vi "CRITERI RICERCA.vi"(6 "banco":i32=2, 8 "collaudi di confronto in":string[](array[string]), 9 "String 2":string="RICERCA COLLAUDI", 10 "Confronti?":bool) -> (0 "ANNULLA":bool=TRUE, 1 "collaudi di confronto":string[](array[string]), 2 "Collaudo selezionato":string, 3 "collaudi confronto descr":string[][](array[string]), 4 "Campi descrittivi confronto":string[](array[string]), 5 "Column Header Strings[]":string[](array[string])=["Banco", "Anno", "Numero", "CODICE", "Data_ora", "Anagrafica_cliente", "TIPO_PRODOTTO", "ARTICOLO", "GENERATORE_marca_generatore", "GENERATORE_marca_motore", "GENERATORE_marca_alternatore", "GENERATORE_matricola_alternatore", "GENERATORE_potenza_KVA", "GENERATORE_tensione_V", "GENERATORE_corrente", "GENERATORE_poli", "GENERATORE_giri", "GENERATORE_frequenza", "GENERATORE_tensione_eccitaz", "GENERATORE_corrente_eccitaz", "GENERICO_marca", "GENERICO_tipo", "GENERICO_matricola", "GENERICO_potenza_kW", "GENERICO_tensione_V", "GENERICO_corrente", "MOTOREac_marca", "MOTOREac_tipo", "MOTOREac_matricola", "MOTOREac_potenza_kW", "MOTOREac_poli", "MOTOREac_tensione_V", "MOTOREac_corrente", "MOTOREeex_marca", "MOTOREeex_tipo", "MOTOREeex_matricola", "MOTOREeex_poli", "MOTOREeex_potenza_kW", "MOTOREeex_tensione_V", "MOTOREeex_corrente", "MOTOREcc_marca", "MOTOREcc_tipo", "MOTOREcc_matricola", "MOTOREcc_potenza", "MOTOREcc_Tensione_Armatura", "MOTOREcc_Corrente_Armatura", "MOTOREcc_Tensione_campo", "MOTOREcc_Corrente_campo", "MOTOREcc_giri", "MOTOREcc_Tensione_dinamo", "POMPA_marca", "POMPA_tipo", "POMPA_matricola", "POMPA_poli", "POMPA_potenza_kw", "POMPA_tensione_V", "POMPA_corrente", "POMPAeex_marca", "POMPAeex_tipo", "POMPAeex_matricola", "POMPAeex_poli", "POMPAeex_potenza_kw", "POMPAeex_tensione_V", "POMPAeex_corrente", "TRASFORM_marca", "TRASFORM_tipo", "TRASFORM_matricola", "TRASFORM_potenza", "TRASFORM_tensione_primario", "TRASFORM_corrente_primario", "TRASFORM_tensione_secondario", "TRASFORM_corrente_secondario", "TRASFORM_gruppo_cei", "TRASFORM_VCC_percentuale", "collaudatore", "notes", "ESITO1", "ESITO2", "ESITO3", "ESITO4", "ESITO5", "ESITO6", "ESITO7", "ESITO8", "ESITO9", "ESITO10", "ESITO11", "ESITO12", "ESITO13", "ESITO14", "ESITO15", "NOTE_collaudo"], 7 "Campo descrittivo collaudo":string)   [LabVIEW 2019]
uses:
  <vilib>/Utility/miscctls.llb/LVRowAndColumnUnsignedTypeDef.ctl
  Global percorso impostazioni.vi
  <vilib>/Utility/file.llb/Read Delimited Spreadsheet (string).vi
  <vilib>/addons/database/Connection.llb/Conn Execute.vi
  <vilib>/addons/database/Recordset.llb/Rec Fetch Recordset Data (R).vi
  <vilib>/Utility/file.llb/Write Delimited Spreadsheet (string).vi
  <vilib>/addons/database/_DB Variant To Data/Database Variant To Data.xnode
  <vilib>/addons/database/NI_Database_API.lvlib
panel:
  in  "ARTICOLO":bool
  in  "TIPO":bool
  in  "CLIENTE":bool
  in  "ARTICOLO":string(combo)="MOTORE C.A."
  in  "TIPO PRODOTTO":string(combo)="3-MOTORE C.A."
  in  "ANAGRAFICA CLIENTE":string(combo)=" "
  out "Boolean":bool
  in  "ORDINA RISULTATI PER:":u16(ring)=5 items=["Banco", "Anno", "Numero", "CODICE", "Data_ora", "Anagrafica_cliente", "TIPO_PRODOTTO", "ARTICOLO", "GENERATORE_marca_generatore", "GENERATORE_marca_motore", "GENERATORE_marca_alternatore", "GENERATORE_matricola_alternatore", "GENERATORE_potenza_KVA", "GENERATORE_tensione_V", "GENERATORE_corrente", "GENERATORE_poli", "GENERATORE_giri", "GENERATORE_frequenza", "GENERATORE_tensione_eccitaz", "GENERATORE_corrente_eccitaz", "GENERICO_marca", "GENERICO_tipo", "GENERICO_matricola", "GENERICO_potenza_kW", "GENERICO_tensione_V", "GENERICO_corrente", "MOTOREac_marca", "MOTOREac_tipo", "MOTOREac_matricola", "MOTOREac_poli", "MOTOREac_potenza_kW", "MOTOREac_tensione_V", "MOTOREac_corrente", "MOTOREac_Frequenza", "MOTOREac_RPMnom", "MOTOREac_RPMmax", "MOTOREac_Costruttore", "MOTOREac_ModelloNr", "MOTOREac_TipoServizio", "MOTOREac_Design", "MOTOREac_ClasseIsol", "MOTOREac_Statore", "MOTOREac_Rotore", "MOTOREac_Note", "MOTOREeex_marca", "MOTOREeex_tipo", "MOTOREeex_matricola", "MOTOREeex_poli", "MOTOREeex_potenza_kW", "MOTOREeex_tensione_V", "MOTOREeex_corrente", "MOTOREcc_marca", "MOTOREcc_tipo", "MOTOREcc_matricola", "MOTOREcc_potenza", "MOTOREcc_Tensione_Armatura", "MOTOREcc_Corrente_Armatura", "MOTOREcc_Tensione_campo", "MOTOREcc_Corrente_campo", "MOTOREcc_giri", "MOTOREcc_Tensione_dinamo", "POMPA_marca", "POMPA_tipo", "POMPA_matricola", "POMPA_poli", "POMPA_potenza_kw", "POMPA_tensione_V", "POMPA_corrente", "POMPAeex_marca", "POMPAeex_tipo", "POMPAeex_matricola", "POMPAeex_poli", "POMPAeex_potenza_kw", "POMPAeex_tensione_V", "POMPAeex_corrente", "TRASFORM_marca", "TRASFORM_tipo", "TRASFORM_matricola", "TRASFORM_potenza", "TRASFORM_tensione_primario", "TRASFORM_corrente_primario", "TRASFORM_tensione_secondario", "TRASFORM_corrente_secondario", "TRASFORM_gruppo_cei", "TRASFORM_VCC_percentuale", "collaudatore", "notes", "ESITO1", "ESITO2", "ESITO3", "ESITO4", "ESITO5", "ESITO6", "ESITO7", "ESITO8", "ESITO9", "ESITO10", "ESITO11", "ESITO12", "ESITO13", "ESITO14", "ESITO15", "NOTE_collaudo"]
  out "transposed array":string[][](array[string])
  in  "Tab Control":T1(tab)=enum."OPZIONI"
  in  "COLLAUDI PER CARICAMENTO":i32(listbox)=-1
  in  "SELEZIONA COLLAUDO":bool
  in  "togli":bool
  in  "Lista collaudi":i32(listbox)=-1
  in  "COLLAUDI DI CONFRONTO":i32(listbox)=-1
  in  "AGGIUNGI CONFRONTO":bool
  in  "Fine":bool
  out "Campo descrittivo":string="Tipologia"
  in  "Scegli campo descrittivo":bool
  in  "Lista campi":i32(listbox)
  in  "salva Criteri":bool
  in  "gestione colonne":bool
  out "String":string
  out "filtri":bool[](array[boolean])=[TRUE, FALSE, FALSE, FALSE, FALSE, FALSE, FALSE]
  out "data":string[][](array[string])=[["1", "20", "1", "0", "", "3-MOTORE C.A.", "MOTORE C.A."], ["1", "20", "2", "0", "", "3-MOTORE C.A.", "MOTORE C.A."], ["1", "20", "3", "0", "", "3-MOTORE C.A.", "MOTORE C.A."], ["1", "20", "4", "0", "", "3-MOTORE C.A.", "MOTORE C.A."], ["1", "20", "5", "0", "", "3-MOTORE C.A.", "MOTORE C.A."], ["1", "20", "6", "0", "", "3-MOTORE C.A.", "MOTORE C.A."], ["1", "20", "7", "0", "", "3-MOTORE C.A.", "MOTORE C.A."], ["1", "20", "8", "0", "", "3-MOTORE C.A.", "MOTORE C.A."], ["1", "20", "9", "0", "", "3-MOTORE C.A.", "MOTORE C.A."], ["1", "20", "10", "0", "", "3-MOTORE C.A.", "MOTORE C.A."], ["1", "20", "11", "0", "", "3-MOTORE C.A.", "MOTORE C.A."], ["1", "20", "12", "0", "", "3-MOTORE C.A.", "MOTORE C.A."], ["1", "20", "13", "0", "", "3-MOTORE C.A.", "MOTORE C.A."], ["1", "20", "14", "0", "", "3-MOTORE C.A.", "MOTORE C.A."], ["1", "20", "15", "0", "", "3-MOTORE C.A.", "MOTORE C.A."], ["1", "20", "16", "0", "", "3-MOTORE C.A.", "MOTORE C.A."], ["1", "20", "17", "0", "", "3-MOTORE C.A.", "MOTORE C.A."], ["1", "20", "18", "0", "", "3-MOTORE C.A.", "MOTORE C.A."], ["1", "20", "19", "0", "", "3-MOTORE C.A.", "MOTORE C.A."], ["1", "20", "20", "0", "", "3-MOTORE C.A.", "MOTORE C.A."], ["1", "20", "21", "0", "", "3-MOTORE C.A.", ""], ["1", "20", "22", "0", "", "3-MOTORE C.A.", ""], ["1", "20", "23", "0", "", "3-MOTORE C.A.", ""], ["1", "20", "24", "0", "", "3-MOTORE C.A.", ""], ["1", "20", "25", "0", "", "3-MOTORE C.A.", ""], ["1", "20", "26", "0", "", "3-MOTORE C.A.", "MOTORE C.A."], ["1", "20", "27", "0", "", "3-MOTORE C.A.", "MOTORE C.A."], ["1", "20", "28", "0", "", "3-MOTORE C.A.", "MOTORE C.A."], ["1", "20", "29", "0", "", "3-MOTORE C.A.", "MOTORE C.A."], ["1", "20", "30", "0", "", "3-MOTORE C.A.", "MOTORE C.A."], ["1", "20", "31", "0", " ", "3-MOTORE C.A.", "MOTORE C.A."], ["1", "20", "32", "0", "", "3-MOTORE C.A.", "MOTORE C.A."], ["1", "20", "33", "0", " ", "3-MOTORE C.A.", "MOTORE C.A."], ["1", "20", "34", "0", " ", "3-MOTORE C.A.", "MOTORE C.A."], ["1", "20", "35", "0", " ", "3-MOTORE C.A.", "MOTORE C.A."], ["1", "20", "36", "0", " ", "3-MOTORE C.A.", "MOTORE C.A."], ["1", "20", "37", "0", " ", "3-MOTORE C.A.", "MOTORE C.A."], ["1", "20", "38", "0", " ", "3-MOTORE C.A.", "MOTORE C.A."], ["1", "20", "39", "0", " ", "3-MOTORE C.A.", "MOTORE C.A."], ["1", "20", "40", "0", " ", "3-MOTORE C.A.", "MOTORE C.A."], ["1", "20", "41", "0", " ", "3-MOTORE C.A.", "MOTORE C.A."], ["1", "20", "42", "0", " ", "3-MOTORE C.A.", "MOTORE C.A."], ["1", "20", "43", "0", " ", "3-MOTORE C.A.", " "], ["1", "20", "44", "0", " ", "3-MOTORE C.A.", " "], ["1", "20", "45", "0", " ", "3-MOTORE C.A.", " "], ["1", "20", "46", "0", " ", "3-MOTORE C.A.", " "], ["1", "20", "47", "0", " ", "3-MOTORE C.A.", " "], ["1", "20", "48", "0", " ", "3-MOTORE C.A.", " "], ["1", "20", "49", "0", " ", "3-MOTORE C.A.", " "], ["1", "20", "50", "0", " ", "3-MOTORE C.A.", " "], ["1", "20", "51", "0", " ", "3-MOTORE C.A.", " "], ["1", "20", "52", "0", "", "3-MOTORE C.A.", ""], ["1", "20", "53", "0", "", "3-MOTORE C.A.", ""], ["1", "20", "54", "0", "", "3-MOTORE C.A.", ""], ["1", "20", "55", "0", "", "3-MOTORE C.A.", ""], ["1", "20", "56", "0", "", "3-MOTORE C.A.", ""], ["1", "21", "1", "0", " ", "3-MOTORE C.A.", " "], ["2", "21", "1", "0", " ", "3-MOTORE C.A.", " "], ["1", "21", "2", "0", " ", "3-MOTORE C.A.", " "], ["1", "21", "3", "0", " ", "3-MOTORE C.A.", " "], ["1", "21", "4", "0", " ", "3-MOTORE C.A.", " "], ["1", "21", "5", "0", " ", "3-MOTORE C.A.", " "], ["2", "21", "2", "0", "", "3-MOTORE C.A.", ""], ["2", "21", "3", "0", "", "3-MOTORE C.A.", ""], ["2", "21", "4", "0", "", "3-MOTORE C.A.", ""], ["2", "21", "5", "0", "", "3-MOTORE C.A.", ""], ["2", "21", "6", "0", "", "3-MOTORE C.A.", ""], ["2", "21", "7", "0", "", "3-MOTORE C.A.", ""], ["2", "21", "8", "0", "", "3-MOTORE C.A.", ""], ["2", "21", "9", "0", "", "3-MOTORE C.A.", ""], ["1", "21", "6", "0", "", "3-MOTORE C.A.", ""], ["1", "21", "7", "0", "", "3-MOTORE C.A.", ""], ["1", "21", "8", "0", "", "3-MOTORE C.A.", ""], ["2", "21", "10", "0", "", "3-MOTORE C.A.", ""], ["2", "21", "12", "0", "", "3-MOTORE C.A.", ""], ["2", "21", "13", "0", "", "3-MOTORE C.A.", ""], ["2", "21", "15", "0", "", "3-MOTORE C.A.", ""], ["2", "21", "14", "0", "", "3-MOTORE C.A.", ""], ["1", "21", "9", "0", "", "3-MOTORE C.A.", "MOTORE C.A."], ["1", "21", "10", "0", "", "3-MOTORE C.A.", "MOTORE C.A."], ["1", "21", "11", "0", "", "3-MOTORE C.A.", "MOTORE C.A."], ["2", "21", "16", "0", "", "3-MOTORE C.A.", ""]]
  in  "aggiorna":bool
  in  "FREQUENZA":string(combo)
  in  "TENSIONE":string(combo)
  in  "H PACCO":string(combo)
  in  "FASI":string(combo)
  in  "MATRICOLA":string(combo)
  in  "TIPO":string(combo)
  in  "MODELLO":string(combo)
  in  "N ORDINE PLP":string(combo)
  in  "ID PROGETTO":string(combo)
  in  "TIPOLOGIA":string(combo)
  in  "CODICE":bool
  in  "CODICE":string(combo)="0"
  in  "NUMERO":bool
  in  "NUMERO":string(combo)="1"
  in  "EXIT":bool
  in  "APPLICA FILTRI":bool
  in  "DATA":bool
  in  "ANNO":bool
  in  "BANCO":bool
  in  "A":timestamp=timestamp(3758775756.541846 s since 1904-01-01) format="%<%H:%M:%S\n%d/%m/%Y>T"
  in  "DA":timestamp=timestamp(3758170956.541846 s since 1904-01-01) format="%<%H:%M:%S\n%d/%m/%Y>T"
  in  "ANNO":string(combo)="23"
  in  "BANCO":string(combo)="2"
  # "DATI GENERALI"
  # "SELEZIONA CAMPO DESCRITTIVO COLLAUDO"
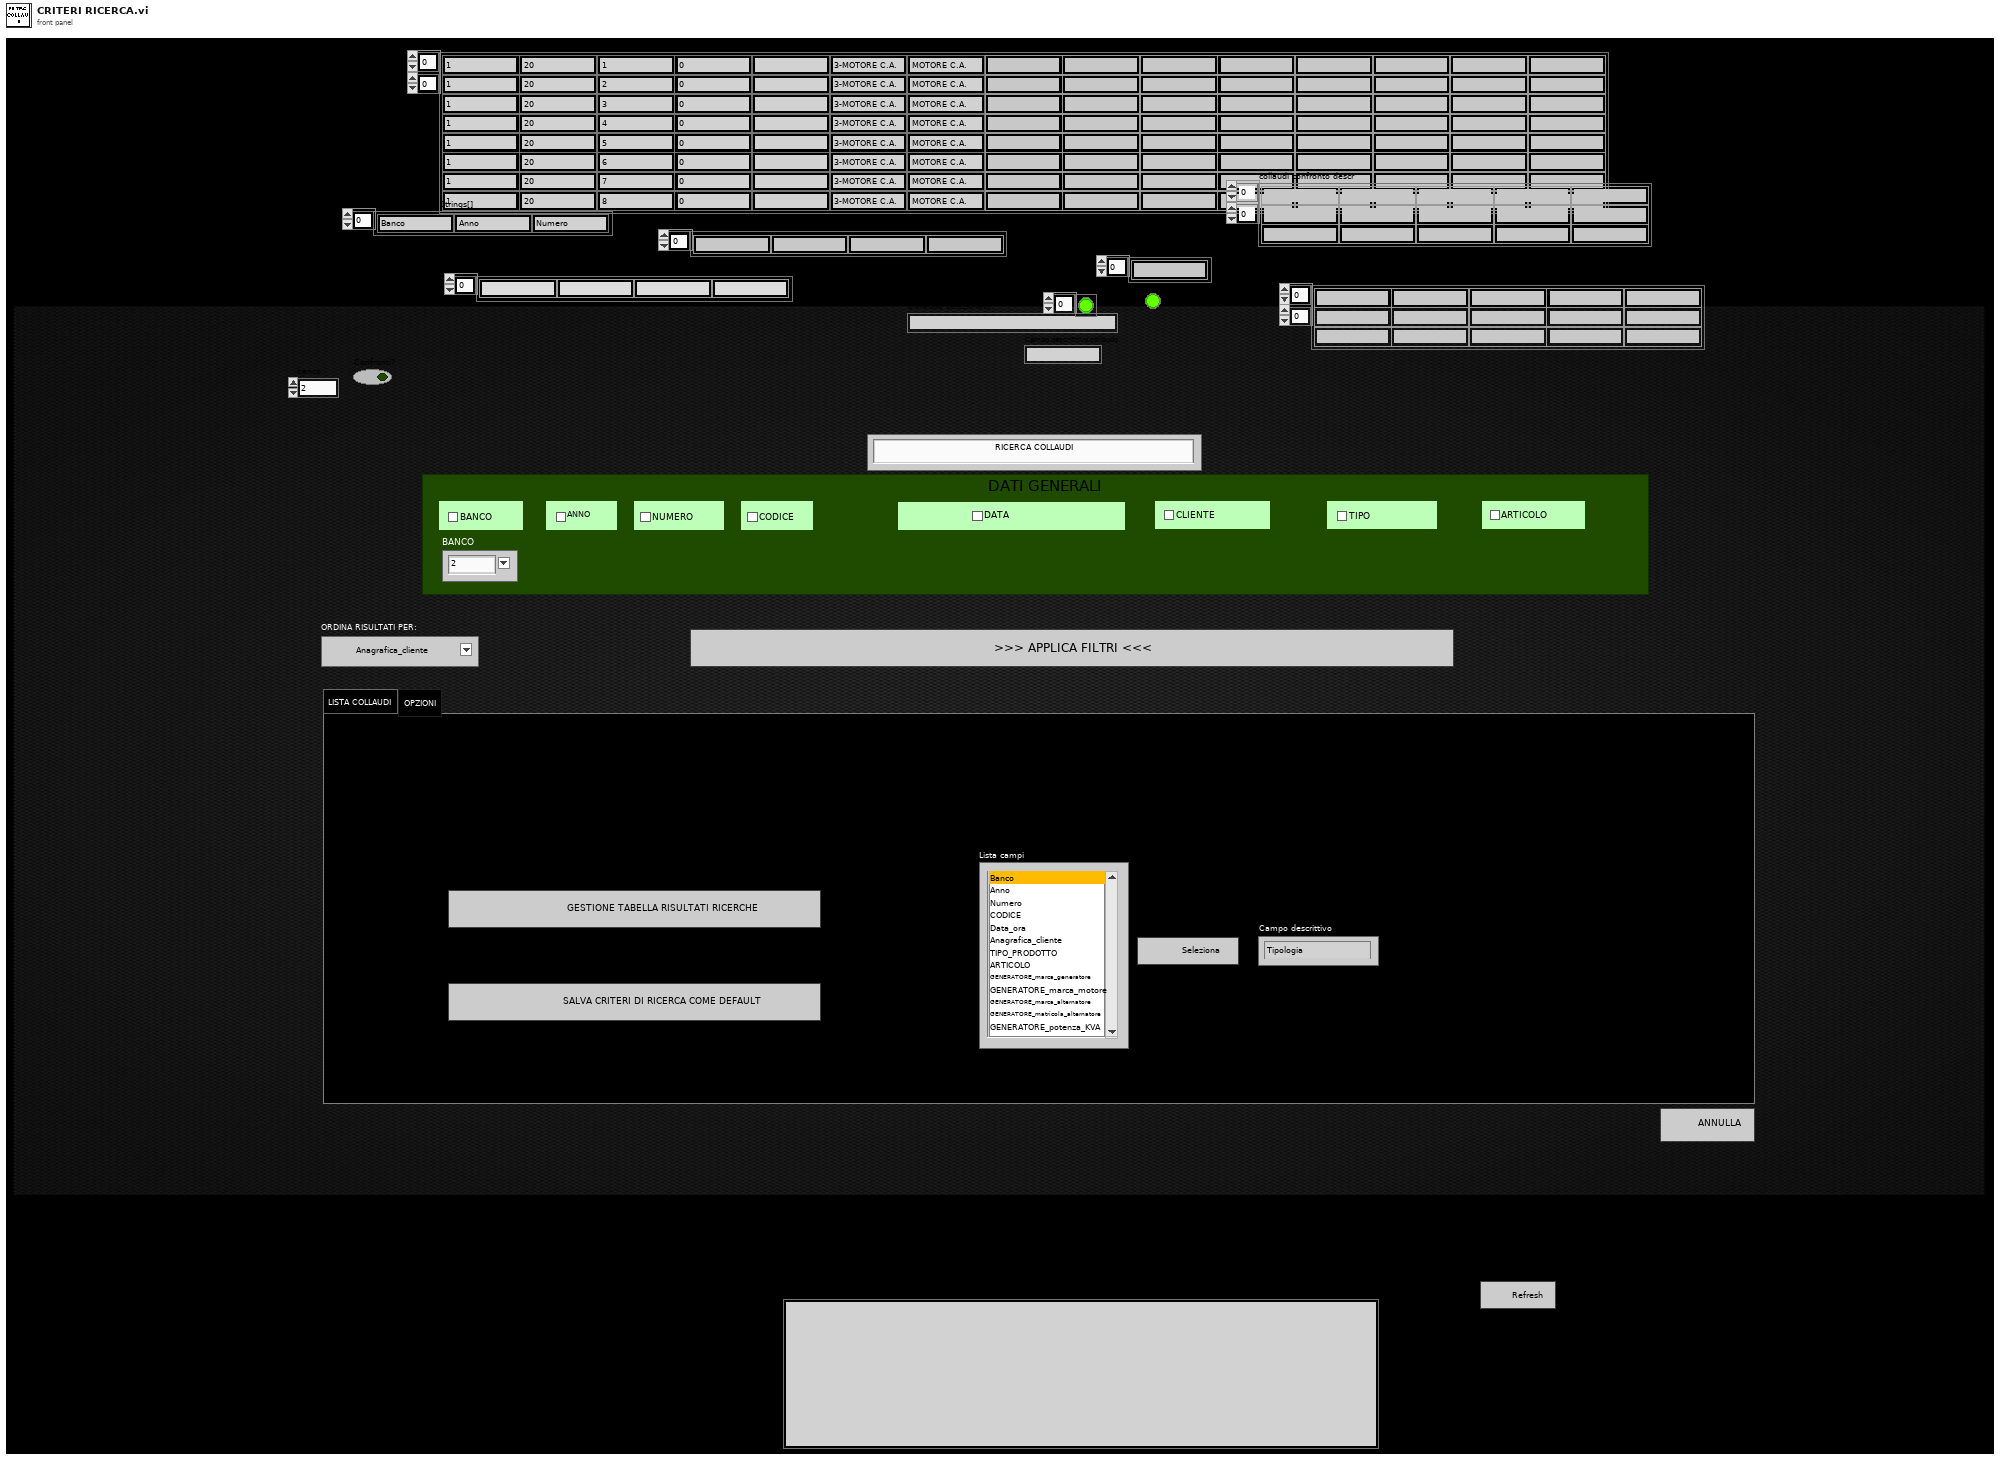
[diagram p1: front panel]
types:
  T1 = enum32{"LISTA COLLAUDI", "COLLAUDI DI CONFRONTO", "OPZIONI"}
  T2 = enum8{"Enabled", "Disabled", "Disabled and Grayed Out"}
  T3 = typedef "LVRowAndColumnUnsignedTypeDef.ctl" = cluster{"Row":u32, "Column":u32}
  T4 = typedef "NI_Database_API.lvlib/Conn ObjectReference.ctl" = refnum<k1>
  T5 = cluster{"index of element":i32, "colonna":string[]}
  T6 = typedef "NI_Database_API.lvlib/Rec ObjectReference.ctl" = refnum<k1>
  T7 = cluster{"index of element":i32, "colonna":string[]}[]
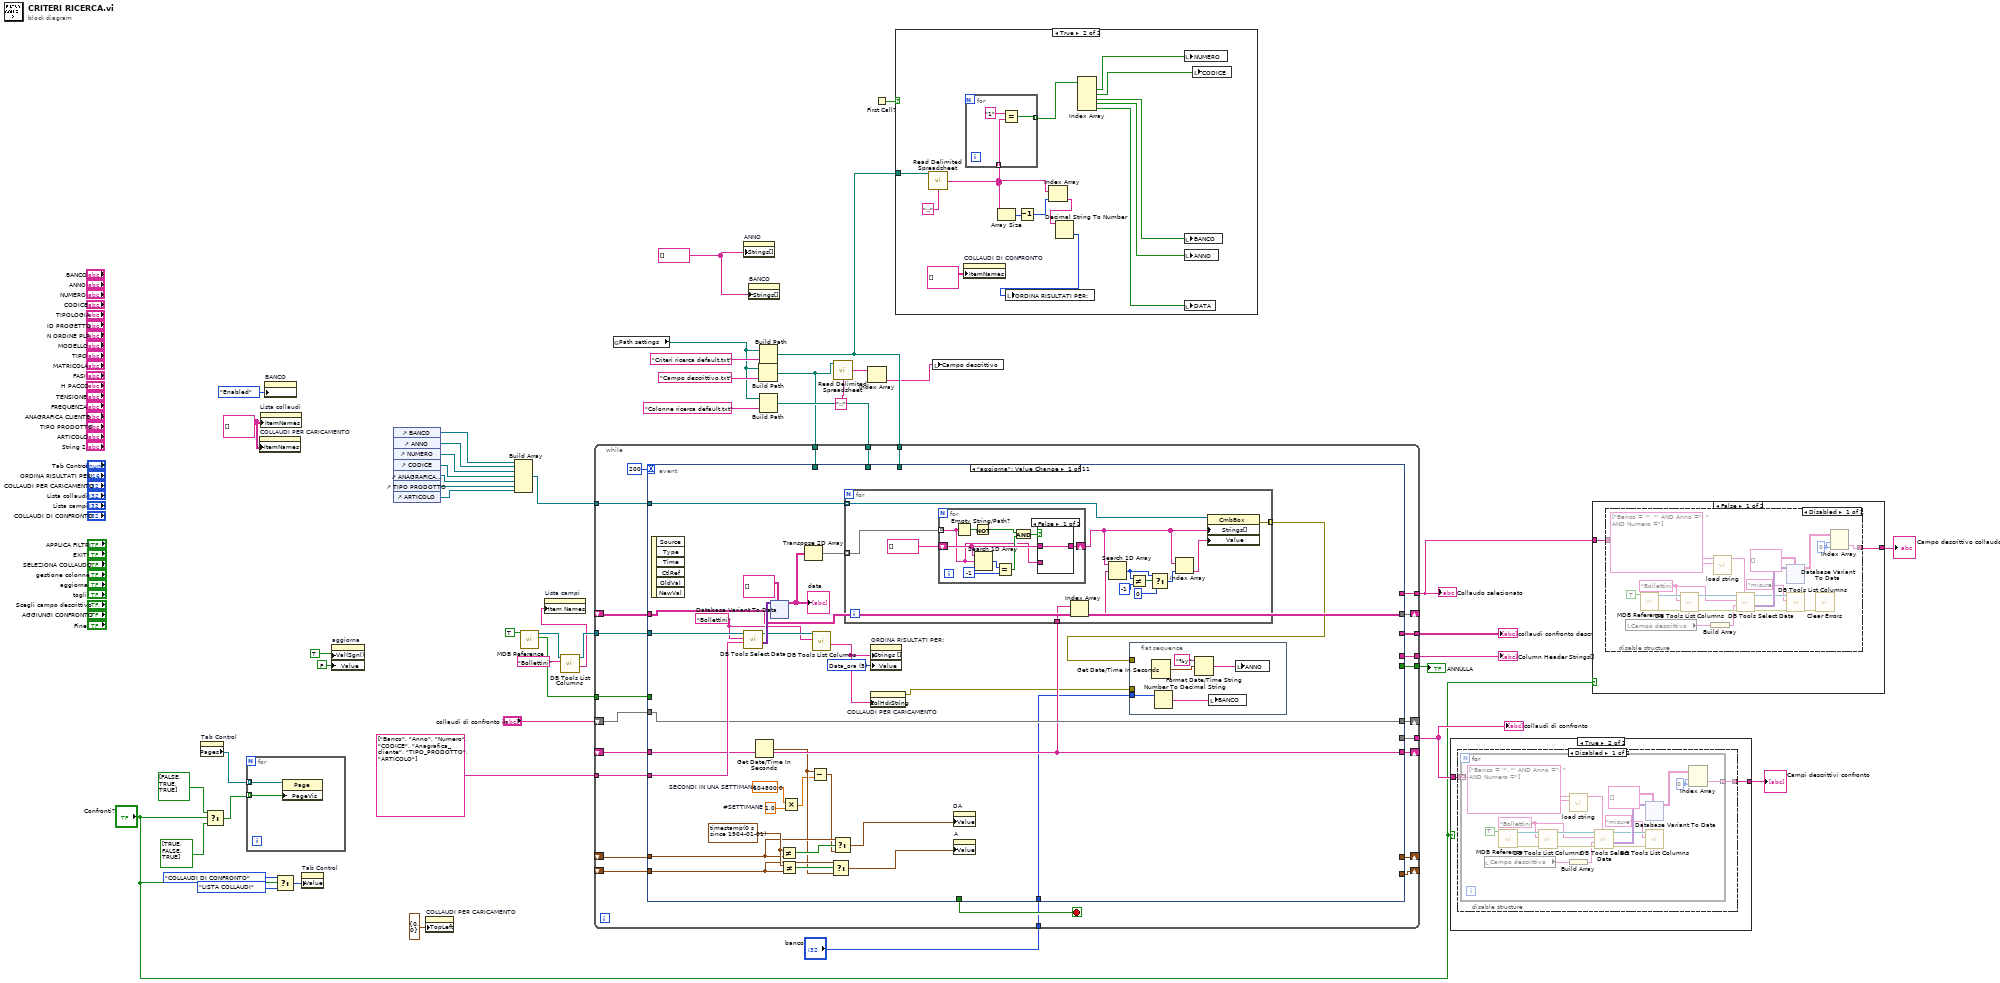
[diagram p0: block diagram]
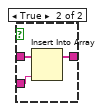
[diagram p7: hidden frame]
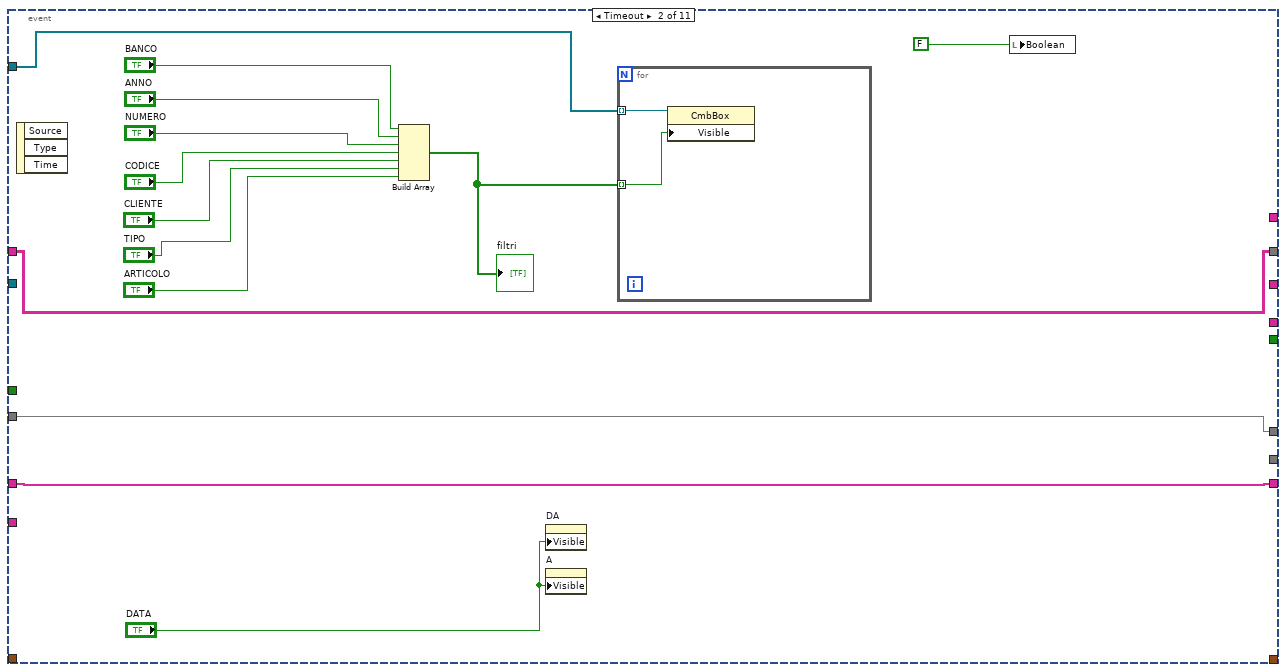
[diagram p8: hidden frame]
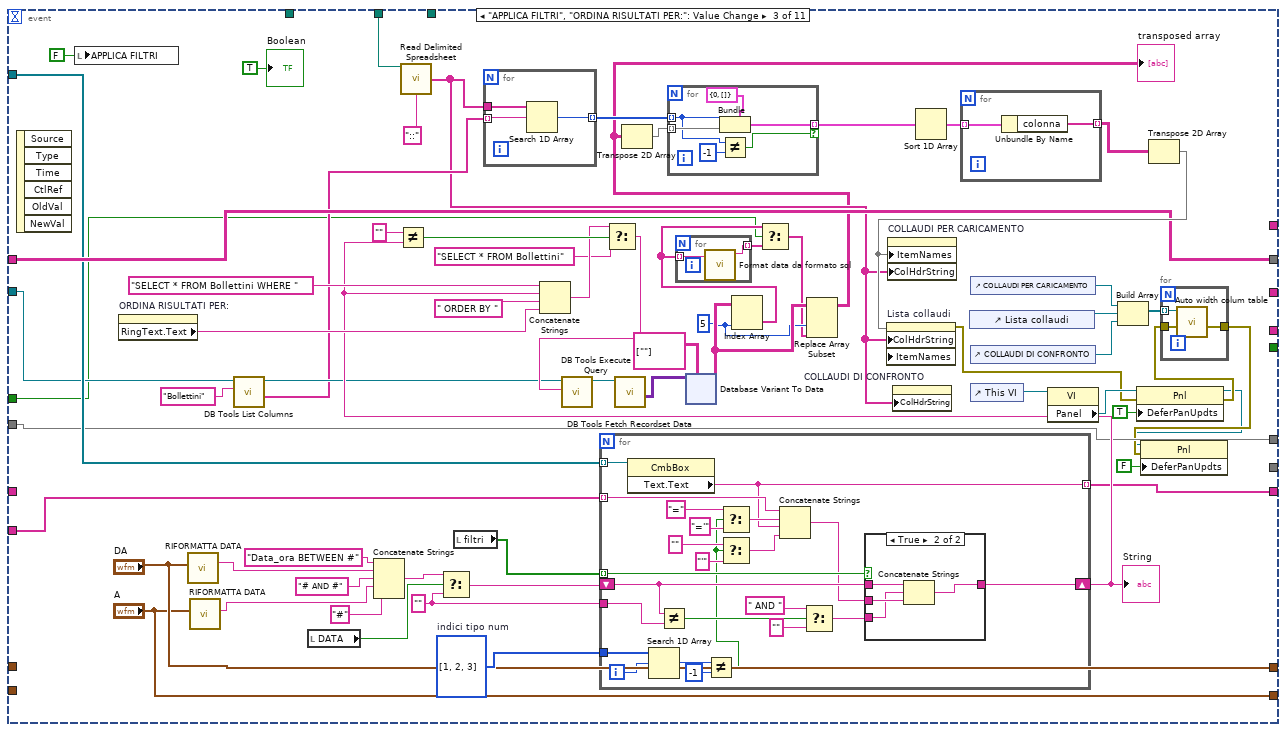
[diagram p9: hidden frame]
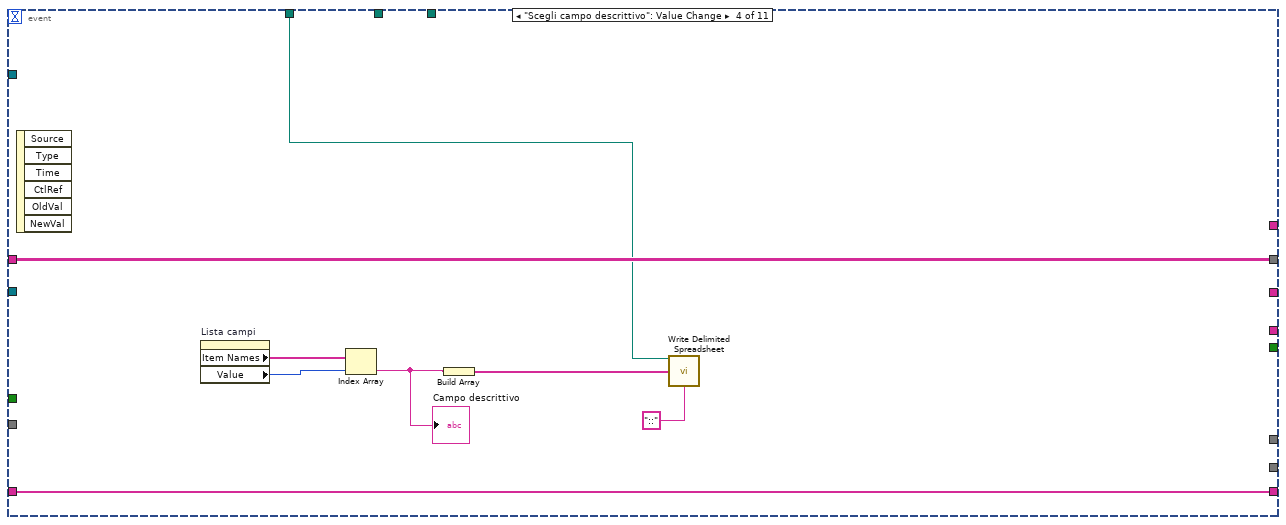
[diagram p11: hidden frame]
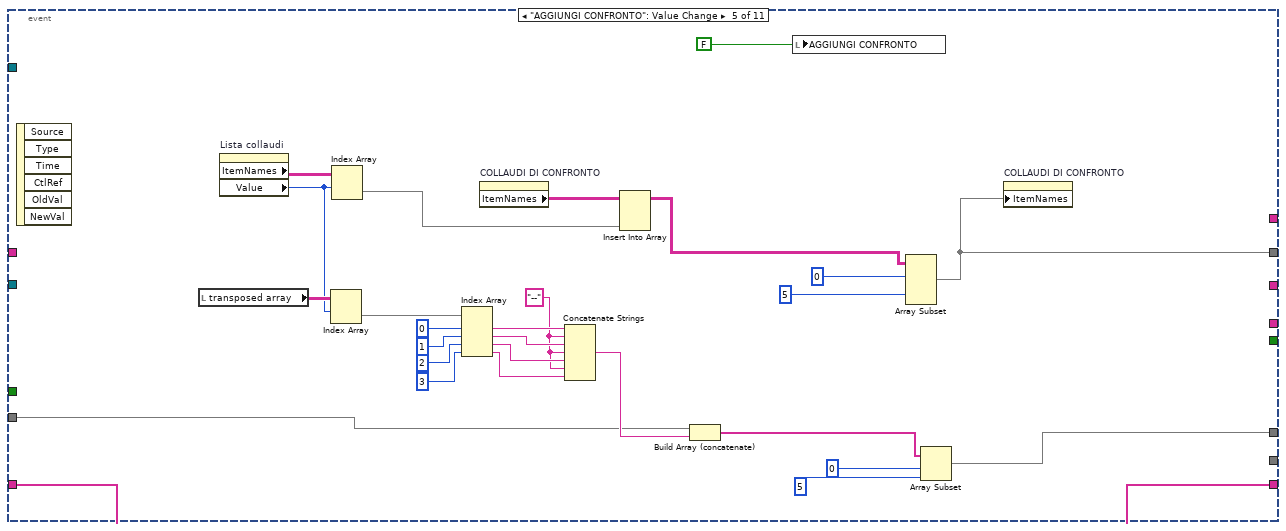
[diagram p12: hidden frame]
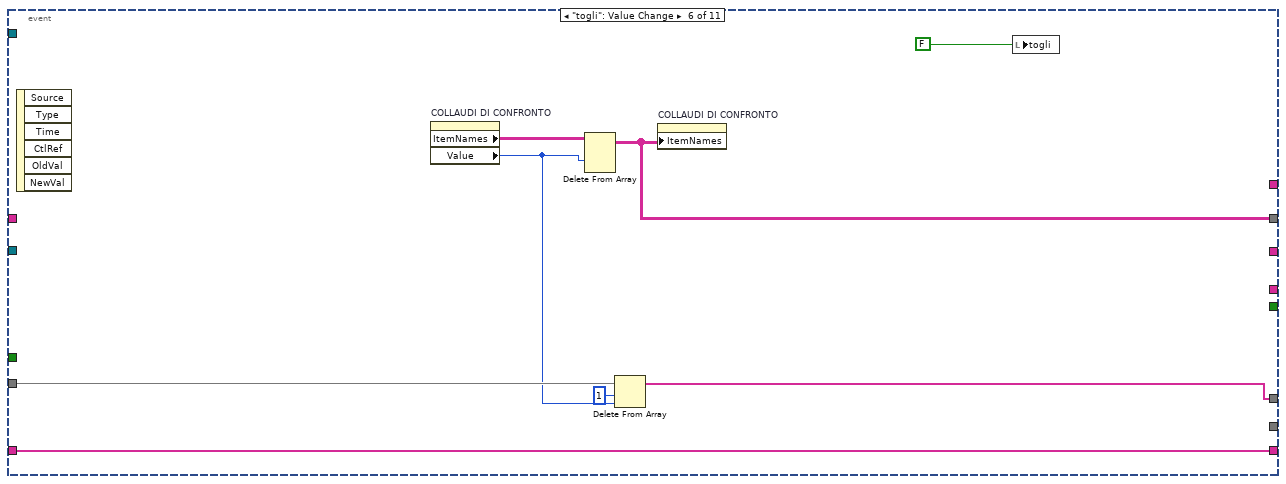
[diagram p13: hidden frame]
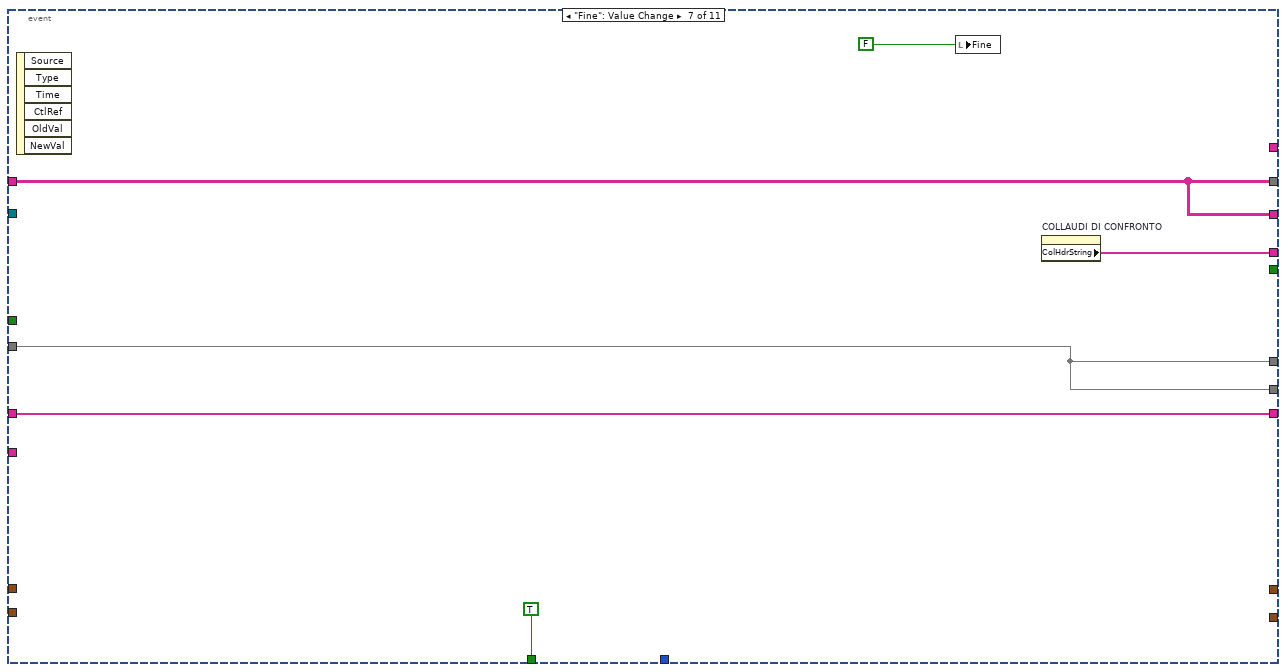
[diagram p14: hidden frame]
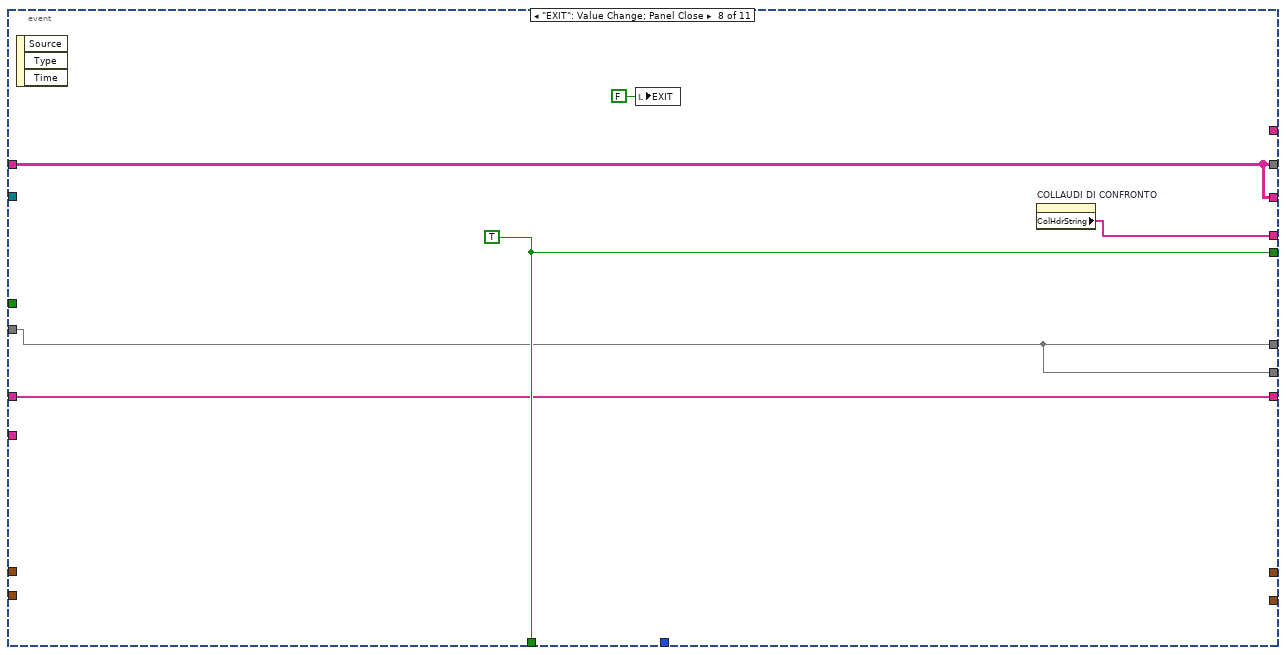
[diagram p15: hidden frame]
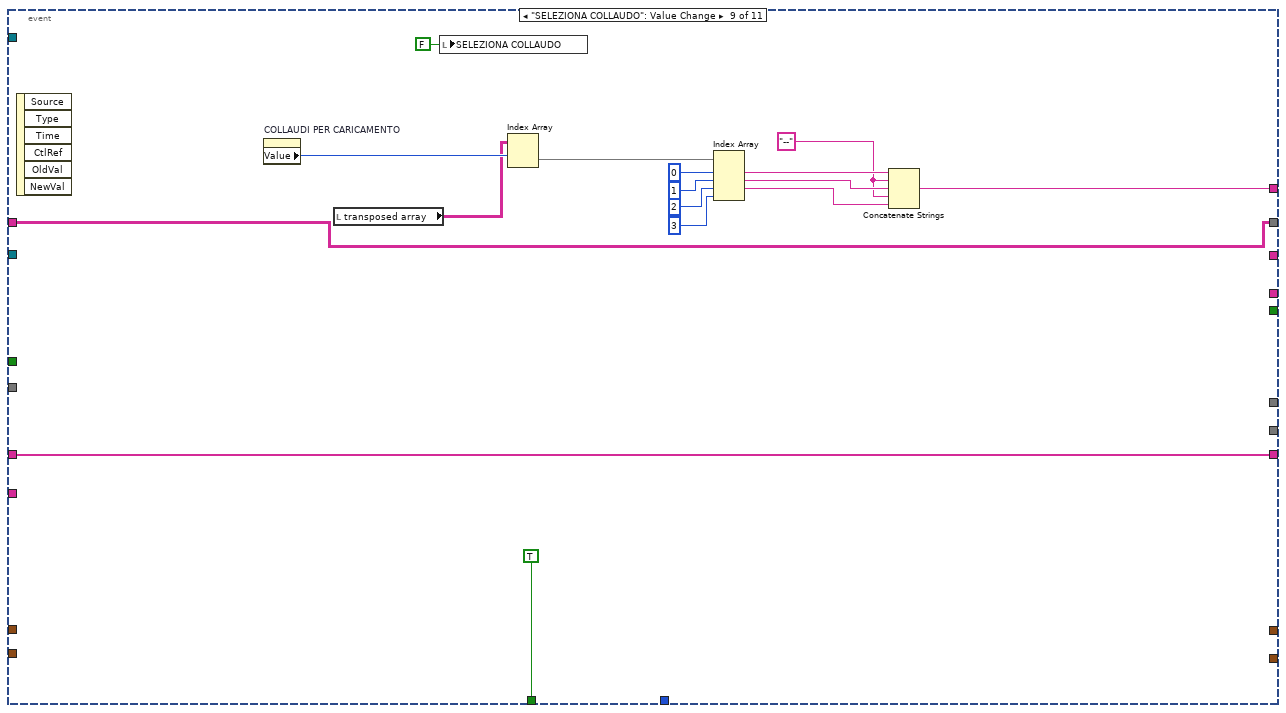
[diagram p16: hidden frame]
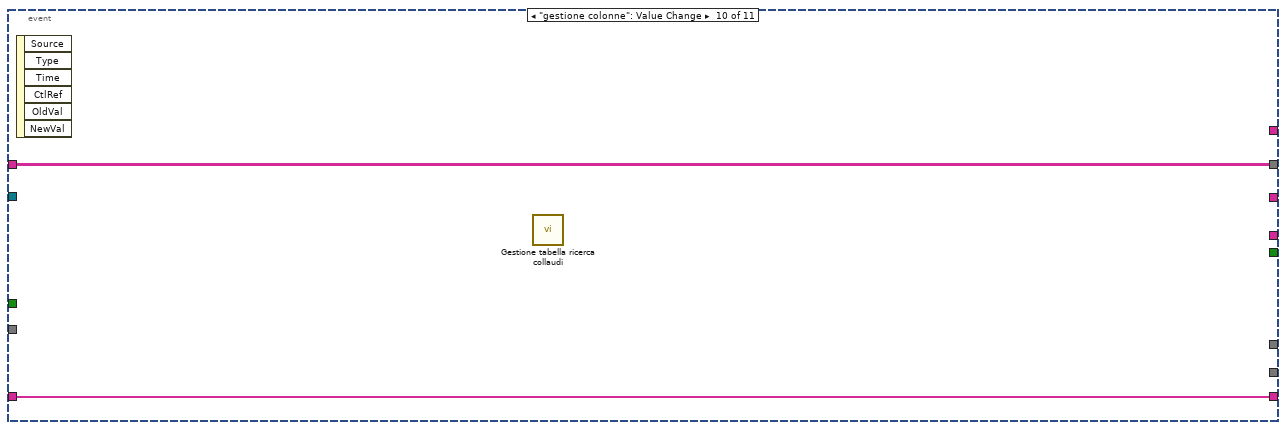
[diagram p17: hidden frame]
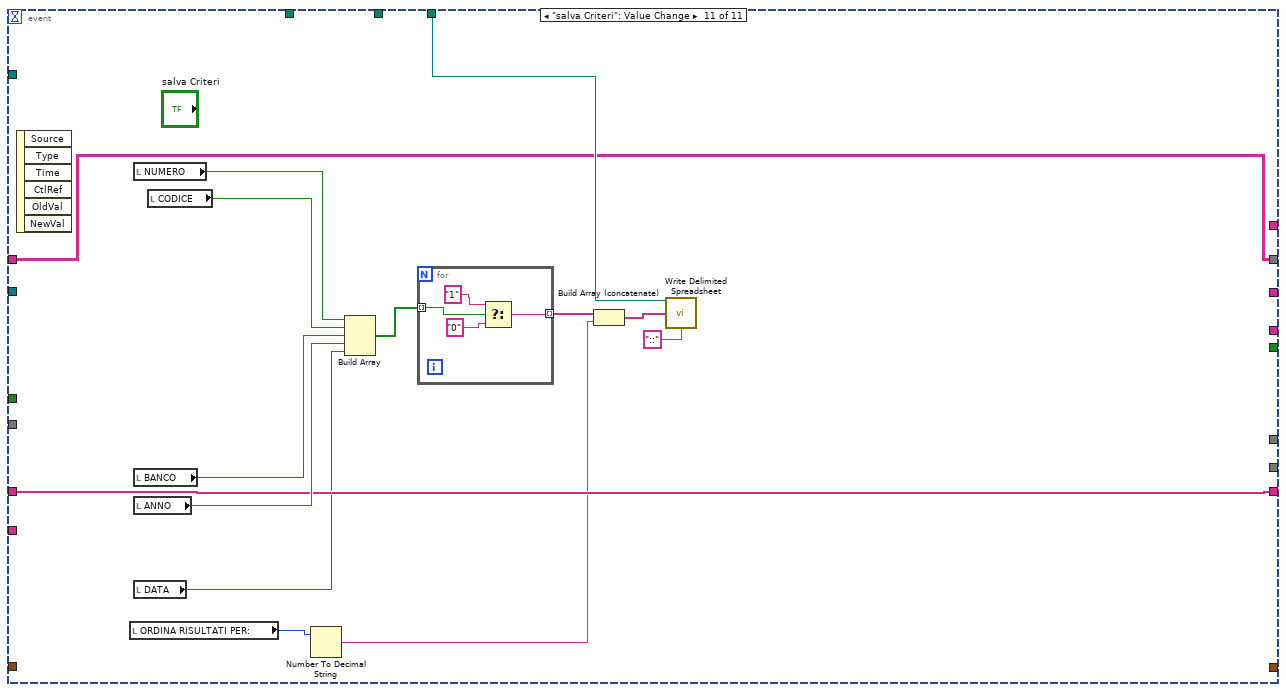
[diagram p18: hidden frame]
diagram:
  w32 = string[][] [] ("Item Names")
  w48 = string[] [] ("Strings []")
  n1 = property on="Tab Control" class="TabCtl (strict)"() -> ("Pages"=w31:refnum<vi>[])  [unwired: 2 in, 2 out]
  n2 = Select(t=bool[] [FALSE, TRUE, TRUE], s="Confronti?", f=bool[] [TRUE, FALSE, TRUE]) -> (s? t:f=w28:bool[])
  n3 = for {
    tunnel: w31 -> [w51] mode=indexing
    tunnel: w28 -> [w50] mode=indexing
    n4 = property class="Page"(reference=w51, "PageVis"=w50) -> ()  [unwired: 1 in, 2 out]
  }
  n5 = property on="COLLAUDI PER CARICAMENTO" class="MCListbox (strict)"("ItemNames"=w32) -> ()  [unwired: 2 in, 2 out]
  n6 = property on="Lista collaudi" class="MCListbox (strict)"("ItemNames"=w32) -> ()  [unwired: 2 in, 2 out]
  n7 = property on="BANCO" class="CmbBox"("DisabledEnum"=T2."Enabled" ("Disabled")) -> ()  [unwired: 2 in, 2 out]
  n8 = Select(t=T1."COLLAUDI DI CONFRONTO" ("Tab Control"), s="Confronti?", f=T1."LISTA COLLAUDI" ("Tab Control")) -> (s? t:f=w25:T1)
  n9 = property on="Tab Control" class="TabCtl (strict)"("Value"=w25) -> ()  [unwired: 2 in, 2 out]
  n10 = property on="aggiorna" class="Bool (strict)"("Val(Sgnl)"=TRUE, "Value"=FALSE ("aggiorna")) -> ()  [unwired: 2 in, 2 out]
  n11 = control-ref of="BANCO"() -> (w46:refnum<vi>)
  n12 = control-ref of="ANNO"() -> (w45:refnum<vi>)
  n13 = control-ref of="NUMERO"() -> (w44:refnum<vi>)
  n14 = control-ref of="CODICE"() -> (w43:refnum<vi>)
  n15 = control-ref of="ANAGRAFICA CLIENTE"() -> (w4:refnum<vi>)
  n16 = control-ref of="TIPO PRODOTTO"() -> (w3:refnum<vi>)
  n17 = control-ref of="ARTICOLO"() -> (w2:refnum<vi>)
  n18 = property on="COLLAUDI PER CARICAMENTO" class="MCListbox (strict)"("TopLeft"=T3 {"Row"=0, "Column"=0} ("Top Left Visible Cell")) -> ()  [unwired: 2 in, 2 out]
  n19 = Build Array(w46, w45, w44, w43, w4, w3, w2) -> (w42:refnum<vi>[])
  n20 = call "MDB Reference.vi"("Collaudi T/motori F"=TRUE ("NM?")) -> ("DB rete(F) Locale(T)"=w20:bool, "Refnum out"=w18:T4)  [unwired: 8 in, 1 out]
  n21 = call <vilib>:"DB Tools List Columns.vi"("table"="Bollettini", "connection reference"=w18) -> ("columns"=w16:string[], "connection reference out"=w17:T4)  [unwired: 2 in, 2 out]
  n22 = property on="Lista campi" class="LstBox (strict)"("Item Names"=w16) -> ()  [unwired: 2 in, 2 out]
  n23 = global read "Global percorso impostazioni.vi" "Path settings"() -> (w12:path)
  n24 = property on="ANNO" class="CmbBox"("Strings[]"=w48) -> ()  [unwired: 2 in, 2 out]
  n25 = property on="BANCO" class="CmbBox"("Strings[]"=w48) -> ()  [unwired: 2 in, 2 out]
  n26 = Build Path(base path=w12, name or relative path="Campo descrittivo.txt") -> (appended path=w10:path)
  n27 = Build Path(base path=w12, name or relative path="Criteri ricerca default.txt") -> (appended path=w37:path)
  n28 = Build Path(base path=w12, name or relative path="Colonne ricerca default.txt") -> (appended path=w36:path)
  n29 = while {
    tunnel: w17 -> [w76]
    tunnel: [w74] -> w7
    tunnel: [w73] -> w47
    tunnel: string[] ["Banco", "Anno", "Numero", "CODICE", "Anagrafica_cliente", "TIPO_PRODOTTO", "ARTICOLO"] ("columns") -> [w72]
    tunnel: w42 -> [w71]
    tunnel: w36 -> [w69]
    tunnel: w37 -> [w68]
    shift-right: [w67] -> _
    shift-left: "collaudi di confronto in" -> [w66]
    tunnel: [w65] -> w15
    shift-right: [w64] -> _
    shift-left: _ -> [w63]
    tunnel: [w62] -> w34
    tunnel: [w61] -> w33
    shift-right: [w60] -> _
    shift-left: _ -> [w59]
    shift-right: [w58] -> _
    shift-left: _ -> [w56]
    shift-right: [w57] -> _
    shift-left: _ -> [w55]
    tunnel: "banco" -> [w54]
    tunnel: w20 -> [w53]
    tunnel: w10 -> [w52]
    stop <- w75 stop-if-true
    n30 = event shown="[0] \"aggiorna\": Value Change" {
      selector: _ -> [_ _ _ _ _ _ _ _ _ _ _]
      dyn-events: _ -> [_ _ _ _ _ _ _ _ _ _ _]
      timeout: 200 -> [_ _ _ _ _ _ _ _ _ _ _]
      tunnel: w76 -> [w103 _ w226 _ _ _ _ _ _ _ _]
      tunnel: [_ _ _ _ _ _ TRUE w404 TRUE _ _] -> w75
      tunnel: [_ _ _ _ _ _ _ _ w411 _ _] -> w74
      tunnel: [_ _ _ _ _ _ _ w404 _ _ _] -> w73
      tunnel: w72 -> [w102 _ w260 _ _ _ _ _ _ _ _]
      tunnel: w71 -> [w99 w191 w234 _ _ _ _ _ _ _ _]
      tunnel: w69 -> [_ _ w229 _ _ _ _ _ _ _ _]
      tunnel: w68 -> [_ _ _ _ _ _ _ _ _ _ w431]
      tunnel: [w95 w188 w233 _ w361 w389 w398 w402 _ _ _] -> w67
      tunnel: w66 -> [w95 w188 w233 _ w369 w391 w398 w402 _ _ _]
      tunnel: [_ _ _ _ _ _ w398 w402 _ _ _] -> w65
      tunnel: [w94 w187 w236 w356 w360 w387 w395 w401 w406 w422 w430] -> w64
      tunnel: w63 -> [w94 w187 w236 w356 _ _ w395 w401 w406 w422 w430]
      tunnel: [_ _ _ _ _ _ w395 w401 _ _ _] -> w62
      tunnel: [_ _ _ _ _ _ w394 w400 _ _ _] -> w61
      tunnel: [w93 w186 w235 w357 w358 w386 w393 w399 w405 w421 w429] -> w60
      tunnel: w59 -> [w93 w186 _ w357 w358 w386 w393 w399 w405 w421 w429]
      tunnel: [_ _ "DA" _ _ _ _ _ _ _ _] -> w58
      tunnel: [_ _ "A" _ _ _ _ _ _ _ _] -> w57
      tunnel: w56 -> [w90 _ _ _ _ _ _ _ _ _ _]
      tunnel: w55 -> [w88 _ _ _ _ _ _ _ _ _ _]
      tunnel: w54 -> [w80 _ _ _ _ _ _ _ _ _ _]
      tunnel: w53 -> [_ _ w198 _ _ _ _ _ _ _ _]
      tunnel: w52 -> [_ _ _ w352 _ _ _ _ _ _ _]
      event "aggiorna": Value Change {
        w78 = u16 5 items=["Banco", "Anno", "Numero", "Tipo_Prova", "Prova_Speciale", "Data_ora", "Norma_rif", "Tipologia", "ID_progetto", "Nordine_PLP", "Rif_cliente", "P_Famiglia", "P_Modello", "P_Matricola", "P_Q1_Lmin", "P_Q2_Lmin", "P_H1", "P_H2", "P_Hmax", "P_Hmin_somm", "P_RPM", "P_Nstadi", "P_DN_mand", "P_DN_asp", "P_Desc_Girante", "P_Desc_Corpo", "M_Modello", "M_Stato", "M_File_Taratura", "M_MEC", "M_Fasi", "M_Hpacco", "M_DN_est_pacco", "M_DN_int_pacco", "M_Tensione", "M_Frequenza", "M_Npoli", "M_RPM", "M_P2_nom", "M_P1_max", "M_Corrente_Max", "M_Rend_Max", "M_CosFi", "M_Condensatore", "M_Classe_isol", "M_Grado_IP", "C_Trasd_PMand", "C_Trasd_PAsp", "C_Dislivello", "C_MisuratoreQ", "C_RapportoTA", "C_Fluido", "C_Temperaura_Fluido", "C_MassaVolumica", "C_Tensione_Vapore", "C_Tamb", "C_Pbarometrica", "C_TensioneProva", "C_FreqProva", "C_Collaudatore", "C_Note", "C_set_Valvole_Tab1", "C_Set_Valvole_Tab2", "C_Set_Valvole_Tab3"] ("ORDINA RISULTATI PER:")
        w82 = 1.0  # #SETTIMANE
        w83 = 604800.0  # SECONDI IN UNA SETTIMANA
        w92 = timestamp(0 s since 1904-01-01) ("DA")
        w97 = "Bollettini" ("table")
        n31 = event-data() -> ()  [unwired: 1 in, 6 out]
        n32 = call <vilib>:"DB Tools Select Data.vi"("columns"=w102, "table"=w97, "connection reference"=w103) -> ("data"=w104:variant[][], "connection reference out"=w98:T4)  [unwired: 3 in, 1 out]
        n33 = Get Date/Time In Seconds() -> (seconds since 1Jan1904=w84:timestamp)
        n34 = xnode "Database Variant To Data"("database variant"=w104, "type"=string[][] [] ("Item Names")) -> ("data"=w101:string[][])  [unwired: 1 in, 1 out]
        "data" <- w101
        n35 = Not Equal?(x=w92, y=w90) -> (x != y?=w91:bool)
        n36 = Not Equal?(x=w92, y=w88) -> (x != y?=w89:bool)
        n37 = Multiply(x=w83, y=w82) -> (x*y=w81:dbl)
        n38 = Transpose 2D Array(2D array=w101) -> (transposed array=w100:string[][])
        n39 = Subtract(x=w84, y=w81) -> (x-y=w85:timestamp)
        n40 = call <vilib>:"DB Tools List Columns.vi"("table"=w97, "connection reference"=w98) -> ("columns"=w96:string[])  [unwired: 2 in, 3 out]
        n41 = Select(t=w88, s=w89, f=w84) -> (s? t:f=w86:timestamp)
        n42 = Select(t=w90, s=w91, f=w85) -> (s? t:f=w87:timestamp)
        n43 = for {
          tunnel: w100 -> [w124] mode=indexing
          tunnel: w99 -> [w123] mode=indexing
          tunnel: w93 -> [w114]
          tunnel: [w111] -> w79 mode=indexing
          i -> [w113]
          n44 = for {
            tunnel: w124 -> [w125] mode=indexing
            shift-right: [w132] -> w120
            shift-left: string[] [] -> [w131]
            n45 = Empty String/Path?(string/path=w125) -> (empty?=w133:bool)
            n46 = Not(x=w133) -> (.not. x?=w127:bool)
            n47 = Search 1D Array(1D array=w131, element=w125) -> (index of element=w130:i32)  [unwired: 1 in]
            n48 = Equal?(x=w130, y=-1) -> (x = y?=w128:bool)
            n49 = And(x=w127, y=w128) -> (x .and. y?=w126:bool)
            n50 = case shown="False" w126 {
              tunnel: [w134 w137] -> w132
              tunnel: w131 -> [w134 w136]
              tunnel: w125 -> [_ w135]
              frame False {
              }
              frame True {
                n51 = Insert Into Array(array=w136, new element=w135) -> (w137:string[])  [unwired: 1 in]
              }
            }
          }
          n52 = Index Array(array=w114, index=w113) -> (element=w112:string)
          n53 = Search 1D Array(1D array=w120, element=w112) -> (index of element=w117:i32)  [unwired: 1 in]
          n54 = Not Equal?(x=w117, y=-1) -> (x != y?=w118:bool)
          n55 = Select(t=w117, s=w118, f=0) -> (s? t:f=w116:i32)
          n56 = Index Array(array=w120, index=w116) -> (element=w121:string)
          n57 = property class="CmbBox"(reference=w123, "Strings[]"=w120, "Value"=w121) -> (error out=w111:errorcluster)  [unwired: 1 in, 1 out]
        }
        n58 = property on="COLLAUDI PER CARICAMENTO" class="MCListbox (strict)"("ColHdrString"=w96) -> (error out=w77:errorcluster)  [unwired: 2 in, 1 out]
        n59 = property on="ORDINA RISULTATI PER:" class="Ring (strict)"("Strings []"=w96, "Value"=w78) -> ()  [unwired: 2 in, 2 out]
        n60 = property on="DA" class="AbsTime (strict)"("Value"=w87) -> ()  [unwired: 2 in, 2 out]
        n61 = property on="A" class="AbsTime (strict)"("Value"=w86) -> ()  [unwired: 2 in, 2 out]
        n62 = flat-sequence {
          tunnel: w80 -> [w106]
          tunnel: w79 -> [_]
          tunnel: w77 -> [_]
          frame #0 {
            n63 = Get Date/Time In Seconds() -> (seconds since 1Jan1904=w108:timestamp)
            n64 = Number To Decimal String(number=w106) -> (decimal integer string=w110:string)  [unwired: 1 in]
            n65 = Format Date/Time String(time format string (%c)="%y", seconds (now)=w108) -> (date/time string=w109:string)  [unwired: 1 in]
            n66 = local write "BANCO"(w110) -> ()
            n67 = local write "ANNO"(w109) -> ()
          }
        }
      }
      event Timeout {
        n68 = event-data() -> ()  [unwired: 1 in, 3 out]
        n69 = Build Array("BANCO", "ANNO", "NUMERO", "CODICE", "CLIENTE", "TIPO", "ARTICOLO") -> (w189:bool[])
        "filtri" <- w189
        n70 = property on="DA" class="AbsTime (strict)"("Visible"="DATA") -> ()  [unwired: 2 in, 2 out]
        n71 = property on="A" class="AbsTime (strict)"("Visible"="DATA") -> ()  [unwired: 2 in, 2 out]
        n72 = for {
          tunnel: w189 -> [w196] mode=indexing
          tunnel: w191 -> [w197] mode=indexing
          n73 = property class="CmbBox"(reference=w197, "Visible"=w196) -> ()  [unwired: 1 in, 2 out]
        }
        n74 = local write "Boolean"(FALSE ("Boolean")) -> ()
      }
      event "APPLICA FILTRI", "ORDINA RISULTATI PER:": Value Change {
        w203 = 5 ("disabled index (col)")
        w245 = i32[] [1, 2, 3]  # indici tipo num
        w247 = "" ("f")
        n75 = event-data() -> ()  [unwired: 1 in, 6 out]
        n76 = local write "APPLICA FILTRI"(FALSE ("APPLICA FILTRI")) -> ()
        n77 = property on="ORDINA RISULTATI PER:" class="Ring (strict)"() -> ("RingText.Text"=w246:string)  [unwired: 2 in, 2 out]
        n78 = call "RIFORMATTA DATA.vi"("time stamp"="DA") -> ("DATA RIFORMATTATA"=w258:string)  [unwired: 10 in]
        n79 = call "RIFORMATTA DATA.vi"("time stamp"="A") -> ("DATA RIFORMATTATA"=w257:string)  [unwired: 10 in]
        n80 = call <vilib>:"DB Tools List Columns.vi"("table"="Bollettini", "connection reference"=w226) -> ("columns"=w224:string[], "connection reference out"=w225:T4)  [unwired: 2 in, 2 out]
        n81 = local read "DATA"() -> (w249:bool)
        n82 = Concatenate Strings("Data_ora BETWEEN #" ("string"), w258, "# AND #" ("string"), w257, "#" ("string")) -> (w254:string)
        n83 = call-poly <vilib>:"Read Delimited Spreadsheet.vi"("file path (dialog if empty)"=w229, "delimiter (\\t)"="::" ("delimiter (\\t)")) -> ("first row"=w218:string[])  [unwired: 8 in, 5 out]
        n84 = Select(t=w254, s=w249, f=w247) -> (s? t:f=w248:string)
        n85 = local read "filtri"() -> (w261:bool[])
        n86 = for {
          tunnel: w224 -> [w277] mode=indexing
          tunnel: [w276] -> w222 mode=indexing
          tunnel: w218 -> [w275]
          n87 = Search 1D Array(1D array=w275, element=w277) -> (index of element=w276:i32)  [unwired: 1 in]
        }
        n88 = for {
          tunnel: w234 -> [w344] mode=indexing
          tunnel: w261 -> [w339] mode=indexing
          tunnel: w260 -> [w343] mode=indexing
          shift-right: [w340] -> w242
          shift-left: w248 -> [w338]
          tunnel: w247 -> [w337]
          tunnel: w245 -> [w327]
          tunnel: [w322] -> w235 mode=indexing
          i -> [w326]
          n89 = property class="CmbBox"(reference=w344) -> ("Text.Text"=w322:string)  [unwired: 1 in, 2 out]
          n90 = Search 1D Array(1D array=w327, element=w326) -> (index of element=w325:i32)  [unwired: 1 in]
          n91 = Not Equal?(x=w338, y=w337) -> (x != y?=w336:bool)
          n92 = Not Equal?(x=w325, y=-1) -> (x != y?=w323:bool)
          n93 = Select(t="=" ("string"), s=w323, f="='" ("string")) -> (s? t:f=w331:string)
          n94 = Select(t="", s=w323, f="'" ("string")) -> (s? t:f=w328:string)
          n95 = Concatenate Strings(w343, w331, w322, w328) -> (w334:string)
          n96 = Select(t=" AND " ("string"), s=w336, f="") -> (s? t:f=w335:string)
          n97 = case shown="True" w339 {
            tunnel: w338 -> [w345 w349]
            tunnel: [w345 w348] -> w340
            tunnel: w335 -> [_ w346]
            tunnel: w334 -> [_ w347]
            frame False {
            }
            frame True {
              n98 = Concatenate Strings(w349, w346, w347) -> (w348:string)
            }
          }
        }
        "String" <- w242
        n99 = Not Equal?(x="", y=w242) -> (x != y?=w243:bool)
        n100 = Concatenate Strings("SELECT * FROM Bollettini WHERE " ("SQL query"), w242, " ORDER BY " ("string"), w246) -> (w240:string)
        n101 = Select(t=w240, s=w243, f="SELECT * FROM Bollettini" ("SQL query")) -> (s? t:f=w239:string)
        n102 = call-poly <vilib>:"DB Tools Execute Query.vi"("SQL query"=w239, "connection reference"=w225) -> ("recordset reference"=w252:T6)  [unwired: 6 in, 1 out]
        n103 = call-poly <vilib>:"DB Tools Fetch Recordset Data.vi"("recordset reference"=w252) -> ("recordset data"=w251:variant[][])  [unwired: 4 in, 2 out]
        n104 = xnode "Database Variant To Data"("database variant"=w251, "type"=string[][] [[""]]) -> ("data"=w204:string[][])  [unwired: 1 in, 1 out]
        n105 = Index Array(array=w204, index (col)=w203) -> (element=w201:string[])  [unwired: 1 in]
        n106 = for {
          tunnel: w201 -> [w263] mode=indexing
          tunnel: [w262] -> w200 mode=indexing
          n107 = call "Format data da formato sql.vi"("aaaa-mm-gg"=w263) -> ("String"=w262:string)  [unwired: 10 in]
        }
        n108 = Select(t=w201, s=w198, f=w200) -> (s? t:f=w202:string[])
        n109 = Replace Array Subset(array=w204, new element=w202, index (col)=w203) -> (w199:string[][])  [unwired: 1 in]
        "transposed array" <- w199
        n110 = Transpose 2D Array(2D array=w199) -> (transposed array=w223:string[][])
        n111 = for {
          tunnel: w223 -> [w274] mode=indexing
          tunnel: w222 -> [w272] mode=indexing
          tunnel: [w273] -> w220 mode=indexing if=w270
          n112 = Bundle(cluster=T5 {"index of element"=0, "colonna"=[]}, "index of element"=w272, "colonna"=w274) -> (w273:T5)
          n113 = Not Equal?(x=w272, y=-1) -> (x != y?=w270:bool)
        }
        n114 = property on="COLLAUDI DI CONFRONTO" class="MCListbox (strict)"("ColHdrString"=w218) -> ()  [unwired: 2 in, 2 out]
        n115 = Sort 1D Array(array=w220) -> (sorted array=w221:T7)
        n116 = for {
          tunnel: w221 -> [w268] mode=indexing
          tunnel: [w267] -> w219 mode=indexing
          n117 = Unbundle By Name(w268) -> ("colonna"=w267:string[])
        }
        n118 = control-ref of="Lista collaudi"() -> (w216:refnum<vi>)
        n119 = control-ref of="COLLAUDI PER CARICAMENTO"() -> (w215:refnum<vi>)
        n120 = control-ref of="COLLAUDI DI CONFRONTO"() -> (w217:refnum<vi>)
        n121 = control-ref of="This VI"() -> (w213:refnum<vi>)
        n122 = property class="VI"(reference=w213) -> ("Panel"=w212:refnum<vi>)  [unwired: 1 in, 2 out]
        n123 = Build Array(w215, w216, w217) -> (w214:refnum<vi>[])
        n124 = Transpose 2D Array(2D array=w219) -> (transposed array=w237:string[][])
        n125 = property on="Lista collaudi" class="MCListbox (strict)"("ColHdrString"=w218, "ItemNames"=w237) -> (error out=w210:errorcluster)  [unwired: 2 in, 1 out]
        n126 = property on="COLLAUDI PER CARICAMENTO" class="MCListbox (strict)"("ItemNames"=w237, "ColHdrString"=w218) -> ()  [unwired: 2 in, 2 out]
        n127 = property class="Pnl"(reference=w212, error in=w210, "DeferPanUpdts"=TRUE ("Defer Panel Updates")) -> (reference out=w206:refnum<vi>, error out=w209:errorcluster)
        n128 = for {
          tunnel: w209 -> [w266]
          tunnel: w214 -> [w265] mode=indexing
          tunnel: [w264] -> w207
          n129 = call "Auto width colum table.vi"("error in (no error)"=w266, "Real Time tabella"=w265) -> ("error out"=w264:errorcluster)  [unwired: 9 in]
        }
        n130 = property class="Pnl"(reference=w206, error in=w207, "DeferPanUpdts"=FALSE ("Defer Panel Updates")) -> ()  [unwired: 2 out]
        "Boolean" <- TRUE ("Boolean")
      }
      event "Scegli campo descrittivo": Value Change {
        n131 = event-data() -> ()  [unwired: 1 in, 6 out]
        n132 = property on="Lista campi" class="LstBox (strict)"() -> ("Item Names"=w355:string[], "Value"=w354:i32)  [unwired: 2 in, 2 out]
        n133 = Index Array(array=w355, index=w354) -> (element=w351:string)
        "Campo descrittivo" <- w351
        n134 = Build Array(w351) -> (w350:string[])
        n135 = call-poly <vilib>:"Write Delimited Spreadsheet.vi"("file path (dialog if empty)"=w352, "1D data"=w350, "delimiter (\\t)"="::" ("delimiter (\\t)")) -> ()  [unwired: 11 in, 2 out]
      }
      event "AGGIUNGI CONFRONTO": Value Change {
        w373 = "--"
        n136 = event-data() -> ()  [unwired: 1 in, 6 out]
        n137 = local read "transposed array"() -> (w382:string[][])
        n138 = property on="Lista collaudi" class="MCListbox (strict)"() -> ("ItemNames"=w384:string[][], "Value"=w381:i32)  [unwired: 2 in, 2 out]
        n139 = Index Array(array=w382, index (row)=w381) -> (element=w371:string[])  [unwired: 1 in]
        n140 = Index Array(array=w384, index (row)=w381) -> (element=w383:string[])  [unwired: 1 in]
        n141 = Index Array(array=w371, index #1=0 ("index"), index #2=1 ("index"), index #3=2 ("index"), index #4=3 ("index")) -> (element #1=w377:string, element #2=w376:string, element #3=w375:string, element #4=w372:string)
        n142 = property on="COLLAUDI DI CONFRONTO" class="MCListbox (strict)"() -> ("ItemNames"=w368:string[][])  [unwired: 2 in, 2 out]
        n143 = Concatenate Strings(w377, w373, w376, w373, w375, w373, w372) -> (w370:string)
        n144 = Insert Into Array(array=w368, new element=w383) -> (w365:string[][])  [unwired: 2 in]
        n145 = Build Array (concatenate)(w369, w370) -> (w362:string[])
        n146 = local write "AGGIUNGI CONFRONTO"(FALSE ("AGGIUNGI CONFRONTO")) -> ()
        n147 = Array Subset(array=w365, index (row)=0 ("index"), length (row)=5 ("length")) -> (w360:string[][])  [unwired: 2 in]
        n148 = Array Subset "Array Subset"(array=w362, index=0, length=5) -> (w361:string[])
        n149 = property on="COLLAUDI DI CONFRONTO" class="MCListbox (strict)"("ItemNames"=w360) -> ()  [unwired: 2 in, 2 out]
      }
      event "togli": Value Change {
        n150 = event-data() -> ()  [unwired: 1 in, 6 out]
        n151 = property on="COLLAUDI DI CONFRONTO" class="MCListbox (strict)"() -> ("ItemNames"=w392:string[][], "Value"=w390:i32)  [unwired: 2 in, 2 out]
        n152 = Delete From Array(array=w392, index (row)=w390) -> (array with subset deleted=w387:string[][])  [unwired: 2 in, 1 out]
        n153 = Delete From Array "Delete From Array"(array=w391, length=1, index=w390) -> (array with subset deleted=w389:string[])  [unwired: 1 out]
        n154 = property on="COLLAUDI DI CONFRONTO" class="MCListbox (strict)"("ItemNames"=w387) -> ()  [unwired: 2 in, 2 out]
        n155 = local write "togli"(FALSE ("togli")) -> ()
      }
      event "Fine": Value Change {
        n156 = event-data() -> ()  [unwired: 1 in, 6 out]
        n157 = local write "Fine"(FALSE ("Fine")) -> ()
        n158 = property on="COLLAUDI DI CONFRONTO" class="MCListbox (strict)"() -> ("ColHdrString"=w394:string[])  [unwired: 2 in, 2 out]
      }
      event "EXIT": Value Change; Panel Close {
        w404 = TRUE
        n159 = event-data() -> ()  [unwired: 1 in, 3 out]
        n160 = local write "EXIT"(FALSE ("EXIT")) -> ()
        n161 = property on="COLLAUDI DI CONFRONTO" class="MCListbox (strict)"() -> ("ColHdrString"=w400:string[])  [unwired: 2 in, 2 out]
      }
      event "SELEZIONA COLLAUDO": Value Change {
        w407 = "--"
        n162 = event-data() -> ()  [unwired: 1 in, 6 out]
        n163 = property on="COLLAUDI PER CARICAMENTO" class="MCListbox (strict)"() -> ("Value"=w420:i32)  [unwired: 2 in, 2 out]
        n164 = local read "transposed array"() -> (w408:string[][])
        n165 = local write "SELEZIONA COLLAUDO"(FALSE ("SELEZIONA COLLAUDO")) -> ()
        n166 = Index Array(array=w408, index (row)=w420) -> (element=w419:string[])  [unwired: 1 in]
        n167 = Index Array(array=w419, index #1=0 ("index"), index #2=1 ("index"), index #3=2 ("index"), index #4=3 ("index")) -> (element #1=w414:string, element #2=w413:string, element #3=w412:string)  [unwired: 1 out]
        n168 = Concatenate Strings(w414, w407, w413, w407, w412) -> (w411:string)
      }
      event "gestione colonne": Value Change {
        n169 = event-data() -> ()  [unwired: 1 in, 6 out]
        n170 = call "Gestione tabella ricerca collaudi.vi"() -> ()  [unwired: 12 in]
      }
      event "salva Criteri": Value Change {
        n171 = event-data() -> ()  [unwired: 1 in, 6 out]
        n172 = local read "ORDINA RISULTATI PER:"() -> (w427:u16)
        n173 = local read "NUMERO"() -> (w424:bool)
        n174 = local read "BANCO"() -> (w436:bool)
        n175 = local read "ANNO"() -> (w435:bool)
        n176 = local read "DATA"() -> (w423:bool)
        n177 = local read "CODICE"() -> (w425:bool)
        n178 = Number To Decimal String(number=w427) -> (decimal integer string=w426:string)  [unwired: 1 in]
        n179 = Build Array(w424, w425, w436, w435, w423) -> (w434:bool[])
        n180 = for {
          tunnel: w434 -> [w439] mode=indexing
          tunnel: [w437] -> w433 mode=indexing
          n181 = Select(t="1", s=w439, f="0") -> (s? t:f=w437:string)
        }
        n182 = Build Array (concatenate)(w433, w426) -> (w428:string[])
        n183 = call-poly <vilib>:"Write Delimited Spreadsheet.vi"("file path (dialog if empty)"=w431, "1D data"=w428, "delimiter (\\t)"="::" ("delimiter (\\t)")) -> ()  [unwired: 11 in, 2 out]
      }
    }
  }
  "Collaudo selezionato" <- w7
  "ANNULLA" <- w47
  "collaudi di confronto" <- w15
  "collaudi confronto descr" <- w34
  "Column Header Strings[]" <- w33
  n184 = call-poly <vilib>:"Read Delimited Spreadsheet.vi"("file path (dialog if empty)"=w10, "delimiter (\\t)"="::" ("delimiter (\\t)")) -> ("first row"=w9:string[])  [unwired: 8 in, 5 out]
  n185 = Index Array(array=w9) -> (element=w8:string)  [unwired: 1 in]
  n186 = First Call?() -> (First Call?: T/F=w24:bool)
  n187 = case shown="True" w24 {
    tunnel: w37 -> [_ w454]
    frame False {
    }
    frame True {
      n188 = call-poly <vilib>:"Read Delimited Spreadsheet.vi"("file path (dialog if empty)"=w454, "delimiter (\\t)"="::" ("delimiter (\\t)")) -> ("first row"=w448:string[])  [unwired: 8 in, 5 out]
      n189 = property on="COLLAUDI DI CONFRONTO" class="MCListbox (strict)"("ItemNames"=string[][] [] ("Item Names")) -> ()  [unwired: 2 in, 2 out]
      n190 = for {
        tunnel: w448 -> [w457] mode=indexing
        tunnel: [w455] -> w452 mode=indexing
        n191 = Equal?(x="1", y=w457) -> (x = y?=w455:bool)
      }
      n192 = Array Size(array=w448) -> (size(s)=w447:i32)
      n193 = Decrement(x=w447) -> (x-1=w446:i32)
      n194 = Index Array(array=w448, index=w446) -> (element=w445:string)
      n195 = Decimal String To Number(string=w445) -> (number=w444:i32)  [unwired: 2 in, 1 out]
      n196 = local write "ORDINA RISULTATI PER:"(w444) -> ()
      n197 = Index Array(array=w452) -> (element #1=w451:bool, element #2=w450:bool, element #3=w443:bool, element #4=w442:bool, element #5=w441:bool)  [unwired: 5 in]
      n198 = local write "NUMERO"(w451) -> ()
      n199 = local write "BANCO"(w443) -> ()
      n200 = local write "ANNO"(w442) -> ()
      n201 = local write "DATA"(w441) -> ()
      n202 = local write "CODICE"(w450) -> ()
    }
  }
  n203 = local write "Campo descrittivo"(w8) -> ()
  n204 = case shown="True" "Confronti?" {
    tunnel: w15 -> [_ w459]
    tunnel: [_ w458] -> w14
    frame False {
    }
    frame True {
      n205 = disable-structure shown="Disabled" {
        disable-tunnel: w459 -> [w461 _]
        disable-tunnel: [w460 _] -> w458
        frame Disabled {
          n206 = for {
            tunnel: w461 -> [w467] mode=indexing
            tunnel: [w464] -> w460 mode=indexing
            w465 = 0 ("disabled index (col)")
            w471 = "Bollettini" ("table")
            n207 = local read "Campo descrittivo"() -> (w463:string)
            n208 = call "MDB Reference.vi"("Collaudi T/motori F"=TRUE ("NM?")) -> ("error out"=w473:errorcluster, "Refnum out"=w475:T4)  [unwired: 8 in, 1 out]
            n209 = call <vilib>:"DB Tools List Columns.vi"("error in (no error)"=w473, "table"=w471, "connection reference"=w475) -> ("error out"=w472:errorcluster, "connection reference out"=w474:T4)  [unwired: 1 in, 2 out]
            n210 = call "load string.vi"("Array in"=string[] ["Banco = '", "' AND Anno =", " AND Numero ="], "Codice"=w467) -> ("String command"=w476:string)  [unwired: 7 in, 2 out]
            n211 = Build Array(w463) -> (w462:string[])
            n212 = call <vilib>:"DB Tools Select Data.vi"("condition"=w476, "error in (no error)"=w472, "columns"=w462, "table"=w471, "connection reference"=w474) -> ("error out"=w470:errorcluster, "data"=w478:variant[][], "connection reference out"=w469:T4)  [unwired: 1 in]
            n213 = xnode "Database Variant To Data"("database variant"=w478, "type"=string[][] [] ("Item Names")) -> ("data"=w466:string[][])  [unwired: 1 in, 1 out]
            n214 = call <vilib>:"DB Tools List Columns.vi"("error in (no error)"=w470, "table"="misure", "connection reference"=w469) -> ()  [unwired: 1 in, 4 out]
            n215 = Index Array(array=w466, index (row)=w465, index (col)=w465) -> (element=w464:string)
          }
        }
        frame Enabled {
        }
      }
    }
  }
  "Campi descrittivi confronto" <- w14
  n216 = case shown="False" "Confronti?" {
    tunnel: w7 -> [w526 _]
    tunnel: [w525 _] -> w5
    frame False {
      n217 = disable-structure shown="Disabled" {
        disable-tunnel: w526 -> [w546 _]
        disable-tunnel: [w528 _] -> w525
        frame Disabled {
          w531 = 0 ("disabled index (col)")
          w536 = "Bollettini" ("table")
          n218 = local read "Campo descrittivo"() -> (w530:string)
          n219 = call "MDB Reference.vi"("Collaudi T/motori F"=TRUE ("NM?")) -> ("error out"=w538:errorcluster, "Refnum out"=w540:T4)  [unwired: 8 in, 1 out]
          n220 = call <vilib>:"DB Tools List Columns.vi"("error in (no error)"=w538, "table"=w536, "connection reference"=w540) -> ("error out"=w537:errorcluster, "connection reference out"=w539:T4)  [unwired: 1 in, 2 out]
          n221 = Build Array(w530) -> (w529:string[])
          n222 = call "load string.vi"("Array in"=string[] ["Banco = '", "' AND Anno =", " AND Numero ="], "Codice"=w546) -> ("String command"=w541:string)  [unwired: 7 in, 2 out]
          n223 = call <vilib>:"DB Tools Select Data.vi"("condition"=w541, "error in (no error)"=w537, "columns"=w529, "table"=w536, "connection reference"=w539) -> ("error out"=w535:errorcluster, "data"=w543:variant[][], "connection reference out"=w534:T4)  [unwired: 1 in]
          n224 = xnode "Database Variant To Data"("database variant"=w543, "type"=string[][] [] ("Item Names")) -> ("data"=w532:string[][])  [unwired: 1 in, 1 out]
          n225 = call <vilib>:"DB Tools List Columns.vi"("error in (no error)"=w535, "table"="misure", "connection reference"=w534) -> ("error out"=w527:errorcluster)  [unwired: 1 in, 3 out]
          n226 = call <vilib>:"Clear Errors.vi"("error in (no error)"=w527) -> ()  [unwired: 5 in, 2 out]
          n227 = Index Array(array=w532, index (row)=w531, index (col)=w531) -> (element=w528:string)
        }
        frame Enabled {
        }
      }
    }
    frame True {
    }
  }
  "Campo descrittivo collaudo" <- w5
